vi "Dashboard Main.vi"() -> ()   [LabVIEW 2014]
uses:
  <vilib>/Rock Robotics/Network Tables/SD Read Boolean.vi
  <vilib>/Rock Robotics/Network Tables/SD Read Number.vi
  <vilib>/Rock Robotics/Network Tables/SD Write Number.vi
  <vilib>/Rock Robotics/Network Tables/SD Read Numeric Array.vi
panel:
  in  "TCP":refnum<k5>
  out "Camera IP":string="172.22.11.2"
  out "Image Message":string="Timeout in Camera Communications"
  in  "Dashboard Tab":enum32{"Drive"}(tab)
  out "Output":string
  in  "SaveImage":bool
  out "Lift Error":bool
  out "Mode":T1(ring)
  out "Mbps 2":bool
  out "Mbps":dbl=0.49174505999856294 format="%#.1g"
  out "fps":dbl=10.0 format="%#.1g"
  in  "Autonomous Selector":u16(ring) items=["No Auto", "Gantry Out", "1 Recycle Bin Drive Left", "Recycle Bin and Tote Drive Left", "1 Tote Drive Right", "Far Can To Feeder Station", "Stop Grabbing My Can"]
  out "Battery Voltage":dbl(knob)=12.13671875 scale=7.0..14.0
  out "CAN Utilization":sgl(graph)=33.08487
  out "CPU Utilization":sgl(graph)=33.93092
  out "Countdown":sgl
  out "Auto Stack Enabled":bool
  out "Tote Count":dbl
  out "Camera Image":T2(plugin-control)
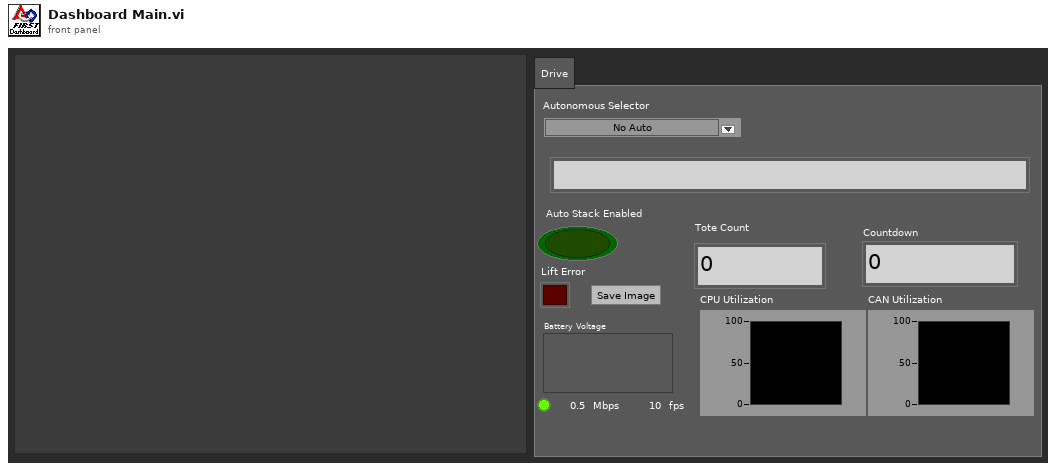
[diagram p1: front panel]
types:
  T1 = enum8{"Tele-Op Disabled", "Tele-Op Enabled", "Auto Disabled", "Auto Enabled", "Test Disabled", "Test Enabled", "Disconnected", "No Code", "E-Stop"}
  T2 = typedef "IMAQ Image.ctl" = refnum<image>
  T3 = enum32{"Drive", "Basic", "Custom", "Test", "Checklist", "Variables"}
  T4 = typedef "Image Type" = u32
  T5 = typedef "Sound Output Task ID.ctl" = u32
  T6 = enum16{"GantrySetpoint", "LiftSetpoint", "ArmSetpoint", "BLSteerError", "BRSteerError", "FLSteerError", "FRSteerError", "GantryError", "LiftLError", "LiftRError", "LeftArmError", "RightArmError"}
  T7 = cluster{"Camera Image":refnum<vi>, "Dashboard Tab":refnum<vi>}
  T8 = cluster{"Frame Rate":i32, "Compression":i32, "Size":u16}
  T9 = cluster{"Error Strings":string, "Disable Counts":cluster{u16, u16}, "Rail Faults":cluster{u16, u16, u16}, "Robot IP":string, "DB Mode":u8, "Event Info":cluster{"Name":string, "Type":u8, "Number":u16, "Replay":u8}, "Camera Addr":string}
  T10 = cluster{"Storage":cluster{"Disk Free":u64, "RAM Block":u32, "RAM free":u32}, "CPU Utilization":cluster{"CPU % ISR":sgl, "CPU % Time Crit":sgl, "CPU % Timed Str":sgl, "CPU % High":sgl, "CPU % Above":sgl, "CPU % Normal":sgl, "CPU % Low":sgl}, "CAN":cluster{"% Bus Utilization":sgl, "Bus Off Cnt":u32, "TX_FIFO Full Cnt":u32, "Receive Error Cnt":u8, "Transmit Error Cnt":u8}, "HID":cluster{"HID Outputs":u32, "Rumble Low":u16, "Rumble High":u16}[]}
  T11 = cluster{"Status bits":cluster{"Test Mode":bool, "Autonomous":bool, "Enabled":bool, "Code Start":bool, "Brownout":bool, "Reserved 2":bool, "Reserved 3":bool, "E-Stop":bool}, "Code Trace":cluster{"Disabled":bool, "TeleOp":bool, "Auto":bool, "Test":bool}, "Controller Type":enum16{"unknown", "cRIO", "roboRio"}, "Code?":enum16{"unknown", "noCode", "code"}, "Battery V":dbl}
  T12 = cluster{"Control Bits":cluster{"TestMode":bool, "Autonomous":bool, "Enabled":bool, "FMS Present":bool, bool, bool, bool, "E-Stop":bool}, "Team Station ":u8, "Countdown":sgl, "Joystick Values":cluster{"Axes":dbl[], "Buttons":bool[], "POVs":i16[]}[]}
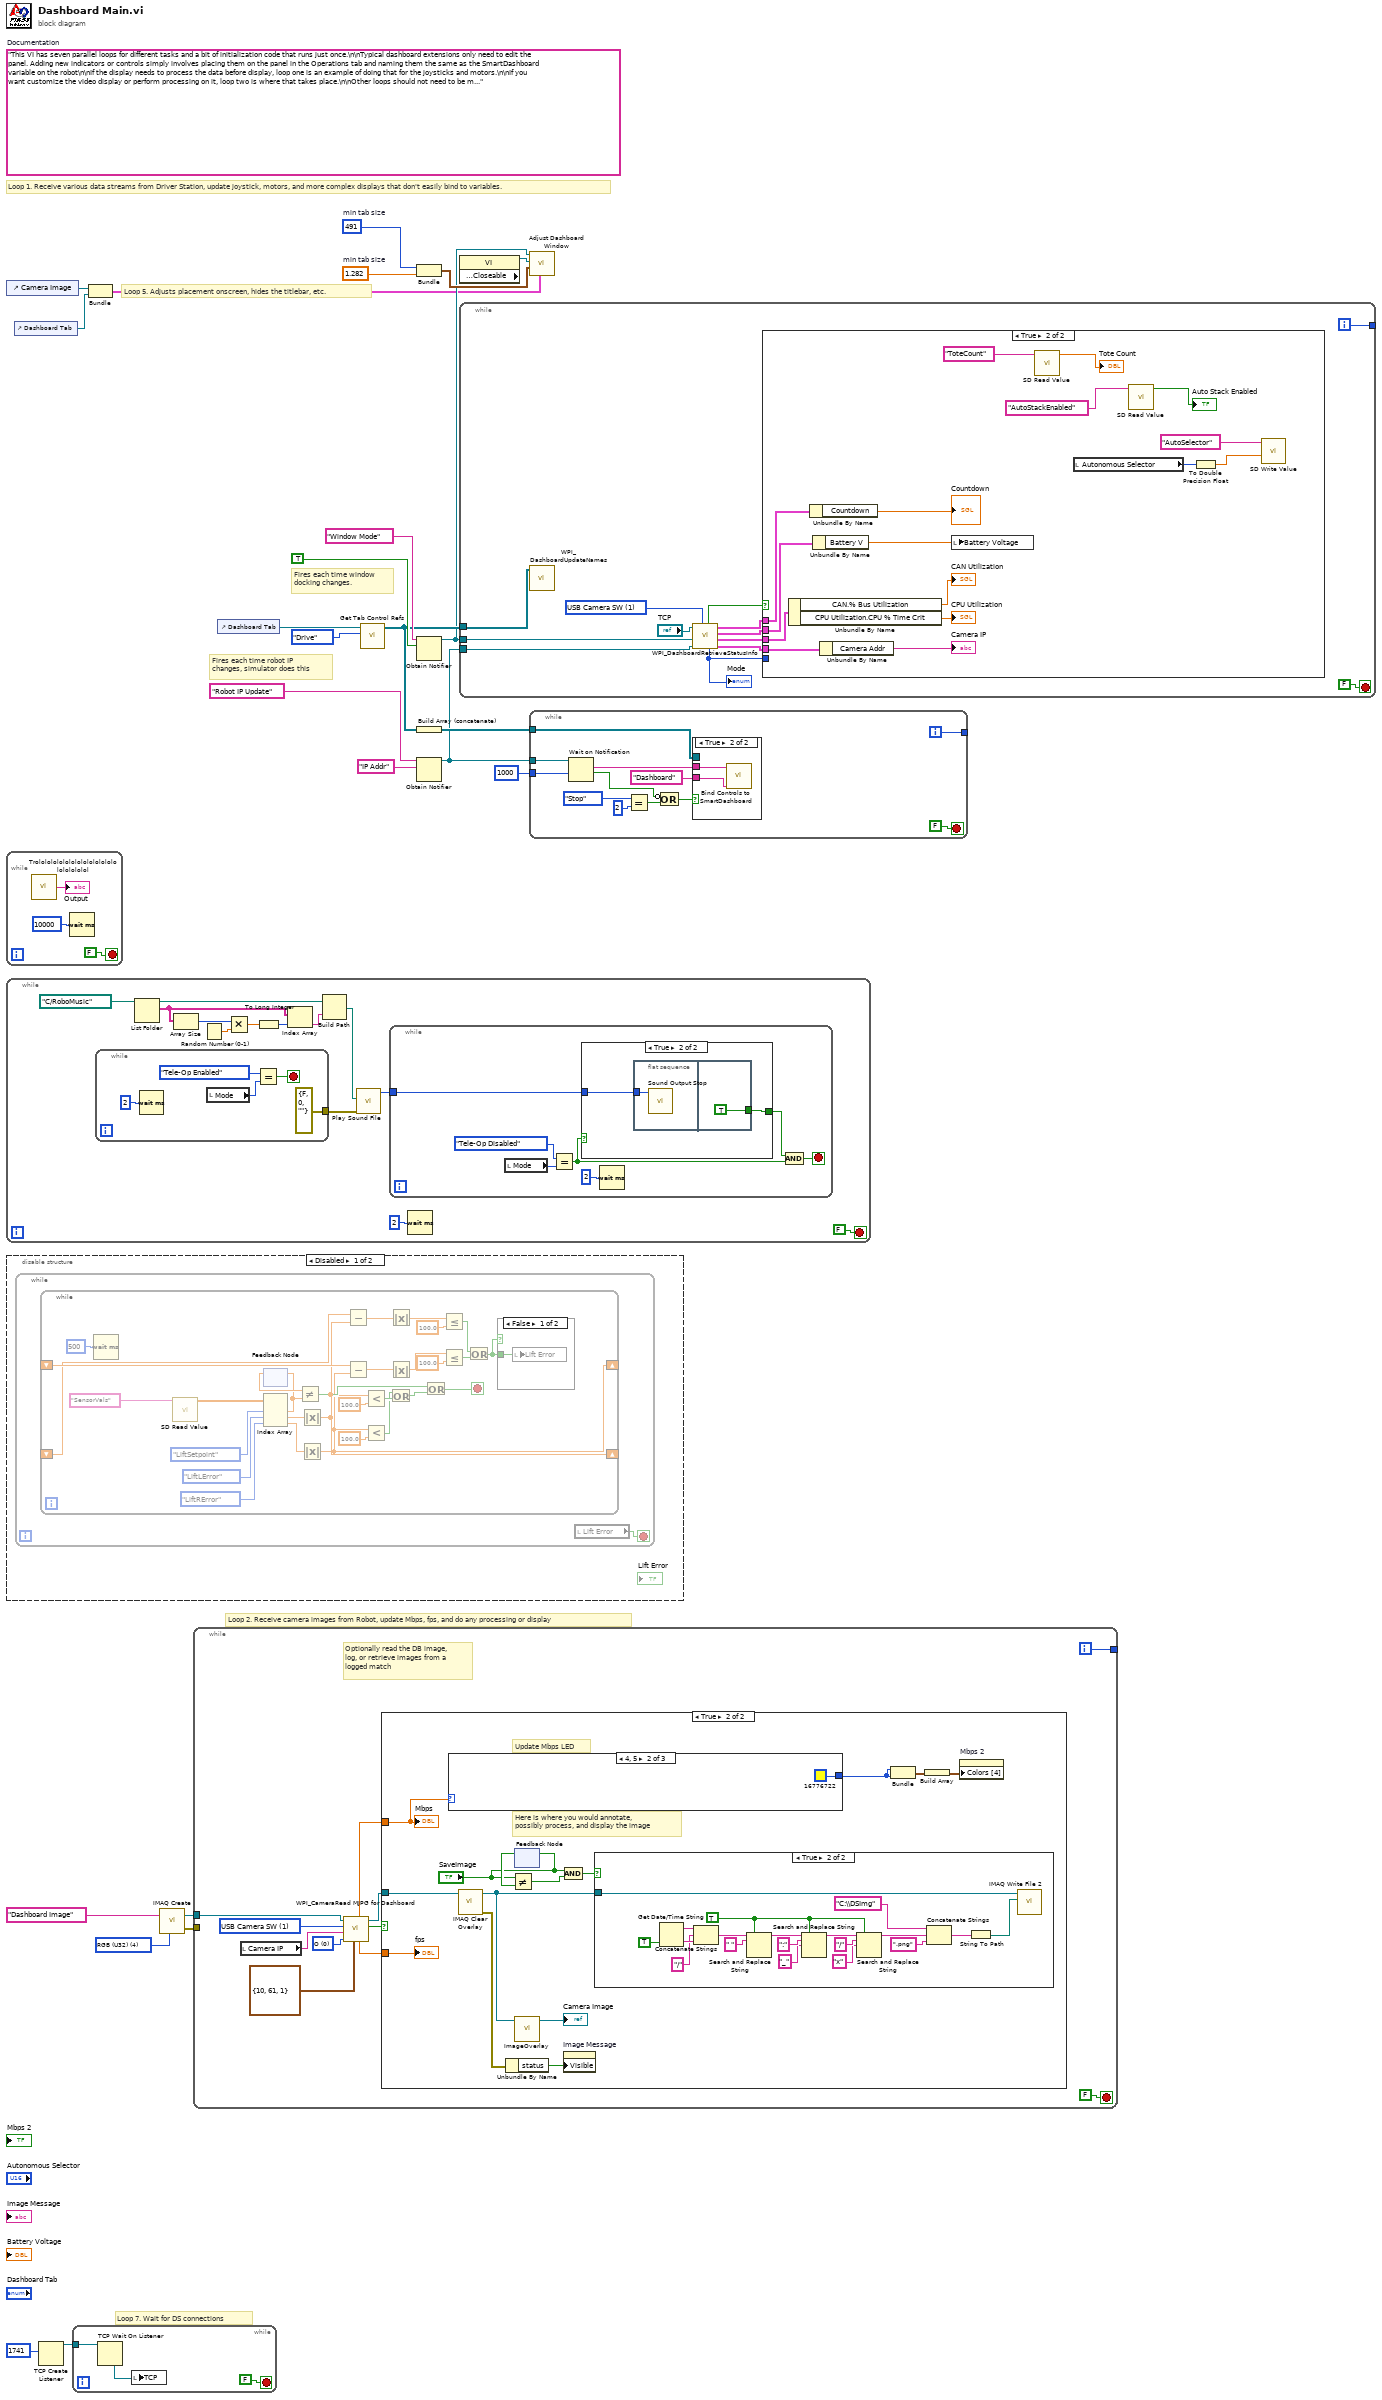
[diagram p0: block diagram]
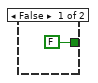
[diagram p2: hidden frame]
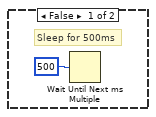
[diagram p7: hidden frame]
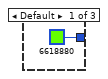
[diagram p9: hidden frame]
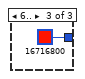
[diagram p10: hidden frame]
diagram:
  w10 = 491  # min tab size
  w9 = 1.282  # min tab size
  (unwired) "This VI has seven parallel loops for different tasks and a bit of initialization code that runs just once.\n\nTypical dashboard extensions only need to edit the panel. Adding new indicators or controls simply involves placing them on the panel in the Operations tab and naming them the same as the SmartDashboard variable on the robot\n\nIf the display needs to process the data before display, loop one is an example of doing that for the joysticks and motors.\n\nIf you want customize the video display or perform processing on it, loop two is where that takes place.\n\nOther loops should not need to be modified. They are pretty standard, and document the task they perform."  # Documentation
  w24 = T4 4 items=["Grayscale (U8)", "Grayscale (I16)", "Grayscale (SGL)", "Complex (CSG)", "RGB (U32)", "HSL (U32)", "RGB (U64)"] ("Image Type")
  # "Loop 7. Wait for DS connections"
  # "Fires each time robot IP\nchanges, simulator does this"
  # "Fires each time window\ndocking changes."
  # "Loop 5. Adjusts placement onscreen, hides the titlebar, etc."
  # "Loop 1. Receive various data streams from Driver Station, update joystick, motors, and more complex displays that don't easily bind to variables."
  # "Loop 2. Receive camera images from Robot, update Mbps, fps, and do any processing or display"
  n1 = control-ref of="Camera Image"() -> (w12:refnum<vi>)
  n2 = while {
    stop <- FALSE stop-if-true
    n3 = call "Trololololololololololololololololololol.vi"() -> ("Message"=→"Output":string)  [unwired: 1 in]
    n4 = Wait (ms)(milliseconds to wait=u32 10000) -> ()  [unwired: 1 out]
  }
  n5 = while {
    stop <- FALSE stop-if-true
    n6 = while {
      tunnel: [errorcluster {"status"=FALSE, "code"=0, "source"=""} ("error in (no error)")] -> w40
      stop <- w55 stop-if-true
      n7 = Wait (ms)(milliseconds to wait=u32 2) -> ()  [unwired: 1 out]
      n8 = local read "Mode"() -> (w57:T1)
      n9 = Equal?(x=T1."Tele-Op Enabled" ("Mode"), y=w57) -> (x = y?=w55:bool)
    }
    n10 = List Folder(path=path "C:/RoboMusic") -> (path out=w30:path, filenames=w31:string[])  [unwired: 3 in, 2 out]
    n11 = Array Size(array=w31) -> (size(s)=w35:i32)
    n12 = Random Number (0-1)() -> (number: 0 to 1=w34:dbl)
    n13 = Multiply(x=w35, y=w34) -> (x*y=w33:dbl)
    n14 = To Long Integer(number=w33) -> (32bit integer=w32:i32)
    n15 = Index Array(array=w31, index=w32) -> (element=w29:string)
    n16 = Build Path(base path=w30, name or relative path=w29) -> (appended path=w28:path)
    n17 = call <vilib>:"Play Sound File.vi"("error in (no error)"=w40, "path"=w28) -> ("task ID"=w39:T5)  [unwired: 8 in, 1 out]
    n18 = while {
      tunnel: w39 -> [w42]
      stop <- w45 stop-if-true
      n19 = local read "Mode"() -> (w46:T1)
      n20 = Equal?(x=T1."Tele-Op Disabled" ("Mode"), y=w46) -> (x = y?=w43:bool)
      n21 = case shown="True" w43 {
        tunnel: [FALSE w50] -> w44
        tunnel: w42 -> [_ w49]
        frame False {
        }
        frame True {
          n22 = flat-sequence {
            tunnel: w49 -> [w51]
            tunnel: [TRUE] -> w50
            frame #0 {
              n23 = call <vilib>:"Sound Output Stop.vi"("task ID"=w51) -> ()  [unwired: 9 in, 2 out]
            }
            frame #1 {
            }
          }
        }
      }
      n24 = Wait (ms)(milliseconds to wait=u32 2) -> ()  [unwired: 1 out]
      n25 = And(x=w44, y=w43) -> (x .and. y?=w45:bool)
    }
    n26 = Wait (ms)(milliseconds to wait=u32 2) -> ()  [unwired: 1 out]
  }
  n27 = disable-structure shown="Disabled" {
    frame Disabled {
      n28 = while {
        stop <- w58 stop-if-true
        n29 = while {
          shift-right: [w65] -> _
          shift-left: _ -> [w66]
          shift-right: [w64] -> _
          shift-left: _ -> [w67]
          stop <- w80 stop-if-true
          n30 = Wait (ms)(milliseconds to wait=u32 500) -> ()  [unwired: 1 out]
          n31 = call-poly <vilib>:"SD Read Value.vi"("Name"="SensorVals") -> ("Numeric Array"=w86:dbl[])  [unwired: 8 in, 2 out]
          n32 = feedback #1() -> (w83:dbl)  [unwired: 1 in]
          n33 = Index Array(array=w86, index #1=T6."LiftSetpoint" ("Enum"), index #2=T6."LiftLError" ("Enum"), index #3=T6."LiftRError" ("Enum")) -> (element #1=w82:dbl, element #2=w78:dbl, element #3=w73:dbl)
          n34 = feedback-in #1(w82) -> ()
          n35 = Not Equal?(x=w83, y=w82) -> (x != y?=w81:bool)
          n36 = Absolute Value(x=w78) -> (abs(x)=w65:dbl)
          n37 = Absolute Value(x=w73) -> (abs(x)=w64:dbl)
          n38 = Subtract(x=w66, y=w65) -> (x-y=w77:dbl)
          n39 = Subtract(x=w67, y=w64) -> (x-y=w69:dbl)
          n40 = Less?(x=w65, y=100.0) -> (x < y?=w72:bool)
          n41 = Less?(x=w64, y=100.0) -> (x < y?=w71:bool)
          n42 = Absolute Value(x=w77) -> (abs(x)=w61:dbl)
          n43 = Absolute Value(x=w69) -> (abs(x)=w60:dbl)
          n44 = Or(x=w71, y=w72) -> (x .or. y?=w70:bool)
          n45 = Or(x=w81, y=w70) -> (x .or. y?=w80:bool)
          n46 = Less Or Equal?(x=w61, y=100.0) -> (x <= y?=w63:bool)
          n47 = Less Or Equal?(x=w60, y=100.0) -> (x <= y?=w62:bool)
          n48 = Or(x=w63, y=w62) -> (x .or. y?=w59:bool)
          n49 = case shown="False" w59 {
            tunnel: w59 -> [w89 _]
            frame False {
              n50 = local write "Lift Error"(w89) -> ()
            }
            frame True {
            }
          }
        }
        n51 = local read "Lift Error"() -> (w58:bool)
      }
    }
    frame Enabled {
    }
  }
  n52 = control-ref of="Dashboard Tab"() -> (w11:refnum<vi>)
  n53 = TCP Create Listener(10:u16 1741 ("timeout ms (25000)")) -> (3:w2:refnum<k5>)  [unwired: 4 in, 2 out]
  n54 = while {
    tunnel: w2 -> [w91]
    stop <- FALSE stop-if-true
    n55 = TCP Wait On Listener(11:w91) -> (4:w90:refnum<k5>)  [unwired: 3 in, 4 out]
    n56 = local write "TCP"(w90) -> ()
  }
  n57 = Bundle("Camera Image"=w12, "Dashboard Tab"=w11) -> (w1:T7)  [unwired: 1 in]
  n58 = call "IMAQ Create"("Image Name"="Dashboard Image", "Image Type"=w24) -> ("New Image"=w22:T2, "error out"=w21:errorcluster)  [unwired: 2 in, 1 out]
  n59 = while {
    tunnel: w22 -> [w101]
    tunnel: w21 -> [_]
    tunnel: [w102] -> _
    i -> [w102]
    stop <- FALSE stop-if-true
    w95 = u16 1 items=["Camera Off", "USB Camera SW", "USB Camera HW", "IP Camera"] ("Vision")
    w93 = u16 0 items=["O", "*", "Open Playback Panel"] ("Rec Mode")
    # "Optionally read the DB image,\nlog, or retrieve images from a\nlogged match"
    n60 = local read "Camera IP"() -> (w94:string)
    n61 = call <vilib>:"WPI_CameraRead MJPG for Dashboard.vi"("Camera Settings"=T8 {"Frame Rate"=10, "Compression"=61, "Size"=1}, "Rec Mode"=w93, "Camera IP"=w94, "Camera Mode"=w95, "Refnum in"=w101) -> ("Active"=w99:bool, "Refnum out"=w100:T2, "FPS"=w98:dbl, "Bandwidth (Mbps)"=w97:dbl)  [unwired: 3 in]
    n62 = case shown="True" w99 {
      tunnel: w100 -> [_ w113]
      tunnel: w97 -> [_ w112]
      tunnel: w98 -> [_ w111]
      frame False {
        # "Sleep for 500ms"
        n63 = Wait Until Next ms Multiple(millisecond multiple=u32 500) -> ()  [unwired: 1 out]
      }
      frame True {
        # "Here is where you would annotate,\npossibly process, and display the image"
        # "Update Mbps LED"
        n64 = case shown="4, 5" w112 {
          tunnel: [u32 6618880 ("Color Box") u32 16776722 ("Color Box") u32 16716800 ("Color Box")] -> w114
          frame Default {
          }
          frame 4, 5 {
          }
          frame 6.. {
          }
        }
        n65 = call "IMAQ Clear Overlay"("Image"=w113) -> ("error out"=w117:errorcluster, "Image Out"=w110:T2)  [unwired: 2 in, 7 out]
        n66 = Unbundle By Name(w117) -> ("status"=w118:bool)
        n67 = feedback #2() -> (w106:bool)  [unwired: 1 in]
        n68 = Not Equal?(x="SaveImage", y=w106) -> (x != y?=w107:bool)
        n69 = feedback-in #2("SaveImage") -> ()
        n70 = call "ImageOverlay.vi"("Refnum in"=w110) -> ("Refnum out"=→"Camera Image":T2)  [unwired: 10 in]
        n71 = And(x="SaveImage", y=w107) -> (x .and. y?=w108:bool)
        n72 = property on="Image Message" class="Str"("Visible"=w118) -> ()  [unwired: 2 in, 2 out]
        n73 = case shown="True" w108 {
          tunnel: w110 -> [_ w137]
          frame False {
          }
          frame True {
            w122 = TRUE ("replace all? (F)")
            n74 = Get Date/Time String(want seconds? (F)=TRUE) -> (date string=w131:string, time string=w121:string)  [unwired: 2 in]
            n75 = Concatenate Strings(w131, "/" ("string"), w121) -> (w132:string)
            n76 = Search and Replace String(replace all?=w122, input string=w132, search string=" ") -> (result string=w129:string)  [unwired: 5 in, 3 out]
            n77 = Search and Replace String(replace all?=w122, input string=w129, search string=":", replace string="_" ("replace string (\"\")")) -> (result string=w126:string)  [unwired: 4 in, 3 out]
            n78 = Search and Replace String(replace all?=w122, input string=w126, search string="/", replace string="x" ("replace string (\"\")")) -> (result string=w125:string)  [unwired: 4 in, 3 out]
            n79 = Concatenate Strings("C:\\DSImg" ("string"), w125, ".png" ("string")) -> (w134:string)
            n80 = String To Path(string=w134) -> (path=w135:path)
            n81 = call-poly "IMAQ Write File 2"("File Path"=w135, "Image"=w137) -> ()  [unwired: 8 in, 2 out]
          }
        }
        n82 = Bundle("Color Box"=w114, "Color Box"=w114) -> (w116:cluster{"Color Box":u32, "Color Box":u32})  [unwired: 1 out]
        n83 = Build Array(w116) -> (w115:cluster{"Color Box":u32, "Color Box":u32}[])
        n84 = property on="Mbps 2" class="Bool (strict)"("Colors [4]"=w115) -> ()  [unwired: 2 in, 2 out]
        "Mbps" <- w112
        "fps" <- w111
      }
    }
  }
  n85 = control-ref of="Dashboard Tab"() -> (w14:refnum<vi>)
  n86 = call <vilib>:"Get Tab Control Refs.vi"("Page Index"=T3."Drive" ("Dashboard Tab"), "TabControl in"=w14) -> ("ControlsOnPage"=w5:refnum<vi>[])  [unwired: 9 in]
  n87 = Bundle("min tab size"=w10, "min tab size"=w9) -> (w8:cluster{"min tab size":i32, "min tab size":dbl})  [unwired: 1 in]
  n88 = Obtain Notifier(name (unnamed)="Window Mode", notification data type=TRUE) -> (notifier out=w4:refnum<notifier>)  [unwired: 2 in, 2 out]
  n89 = Build Array (concatenate)(w5) -> (w13:refnum<vi>[])
  n90 = Obtain Notifier(name (unnamed)="Robot IP Update", notification data type="IP Addr" ("name (unnamed)")) -> (notifier out=w6:refnum<notifier>)  [unwired: 2 in, 2 out]
  n91 = property class="VI" props=["Front Panel.Closeable"]() -> (reference out=w15:refnum<vi>)  [unwired: 2 in, 2 out]
  n92 = while {
    tunnel: [w152] -> _
    tunnel: w6 -> [w146]
    tunnel: w5 -> [w145]
    tunnel: w4 -> [w142]
    i -> [w152]
    stop <- FALSE stop-if-true
    w141 = u16 1 items=["Camera Off", "USB Camera SW", "USB Camera HW", "IP Camera"] ("Vision")
    n93 = call <vilib>:"WPI_DashboardUpdateNames.vi"("Controls on Tab"=w145) -> ()  [unwired: 11 in]
    n94 = call <vilib>:"WPI_DashboardRetrieveStatusInfo.vi"("Vision"=w141, "Binding Refnum"=w146, "Window Mode Notifier"=w142, "TCP Cnx"="TCP") -> ("Power and Errors"=w147:T9, "Robot Metrics"=w150:T10, "Status Info"=w151:T11, "Control Info"=w148:T12, "Robot Mode"=w144:T1, "Process?"=w149:bool)  [unwired: 2 in]
    "Mode" <- w144
    n95 = case shown="True" w149 {
      tunnel: w151 -> [_ w164]
      tunnel: w150 -> [_ w162]
      tunnel: w148 -> [_ w159]
      tunnel: w147 -> [_ w169]
      tunnel: w144 -> [_ _]
      frame False {
      }
      frame True {
        n96 = Unbundle By Name(w162) -> ("CAN.% Bus Utilization"=→"CAN Utilization":sgl, "CPU Utilization.CPU % Time Crit"=→"CPU Utilization":sgl)
        n97 = Unbundle By Name(w159) -> ("Countdown"=→"Countdown":sgl)
        n98 = Unbundle By Name(w164) -> ("Battery V"=w163:dbl)
        n99 = Unbundle By Name(w169) -> ("Camera Addr"=→"Camera IP":string)
        n100 = local write "Battery Voltage"(w163) -> ()
        n101 = call-poly <vilib>:"SD Read Value.vi"("Name"="ToteCount") -> ("Numeric"=→"Tote Count":dbl)  [unwired: 8 in, 2 out]
        n102 = local read "Autonomous Selector"() -> (w165:u16)
        n103 = call-poly <vilib>:"SD Read Value.vi"("Name"="AutoStackEnabled") -> ("Boolean"=→"Auto Stack Enabled":bool)  [unwired: 8 in, 2 out]
        n104 = To Double Precision Float(number=w165) -> (double precision float=w167:dbl)
        n105 = call-poly <vilib>:"SD Write Value.vi"("Numeric"=w167, "Name"="AutoSelector") -> ()  [unwired: 8 in, 2 out]
      }
    }
  }
  n106 = call "Adjust Dashboard Window.vi"("Sizing Refnums"=w1, "Size Constraints"=w8, "VI"=w15, "Notifier in"=w4) -> ()  [unwired: 8 in]
  n107 = while {
    tunnel: w13 -> [w181]
    tunnel: w6 -> [w179]
    tunnel: [w177] -> _
    tunnel: u32 1000 ("milliseconds to wait") -> [w176]
    i -> [w177]
    stop <- FALSE stop-if-true
    n108 = Wait on Notification(notifier=w179, timeout in ms (-1)=w176) -> (notification=w178:string, timed out?=w174:bool)  [unwired: 2 in, 2 out]
    n109 = Equal?(x=enum32{"Stop", "Record", "Playback"}."Stop" ("Rec Mode"), y=u16 2 ("Rec Mode")) -> (x = y?=w173:bool)
    n110 = Compound Arithmetic op=OR(invert w174, w173) -> (w175:bool)
    n111 = case shown="True" w175 {
      tunnel: w181 -> [_ _]
      tunnel: w178 -> [_ w183]
      tunnel: "Dashboard" -> [_ w182]
      frame False {
      }
      frame True {
        n112 = call <vilib>:"Bind Controls to SmartDashboard.vi"("Client Name"=w182, "Server IP Address"=w183) -> ()  [unwired: 10 in]
      }
    }
  }
